vi "Select State(s)_err.vi"(0 "State(s) if True (\"\")":string, 5 "Select":errorcluster, 7 "State(s) if False (\"\")":string) -> (6 "States Out":string)   [LabVIEW 2013]
doc: "Passes State(s) based on a condition\n\nFor instructions on how to use the JKI State Machine, examples and video tutorials, visit:\nhttp://jkisoft.com/state-machine/"
panel:
  # "For instructions on how to use the JKI State Machine, examples and video tutorials, visit:\nhttp://jki.net/state-machine/\n\nJKI State Machine™\nhttp://jki.net/state-machine/\nCopyright (C) 2005-2024, JKI <info@jki.net>\nALL RIGHTS RESERVED"
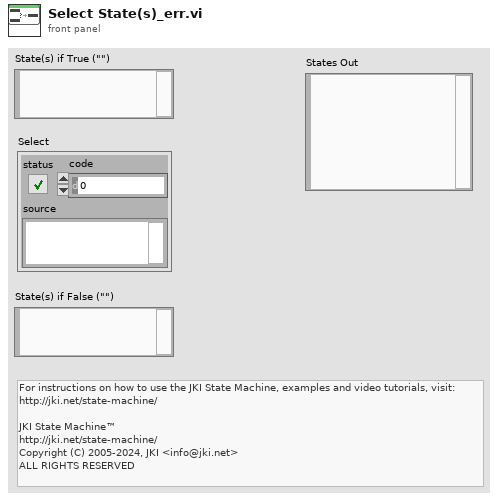
[diagram p1: front panel]
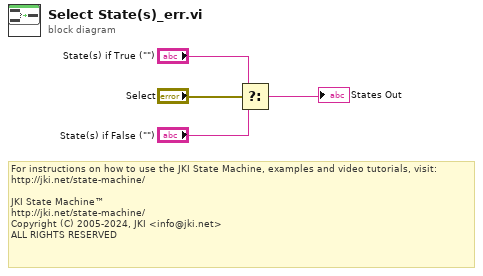
[diagram p0: block diagram]
diagram:
  # "For instructions on how to use the JKI State Machine, examples and video tutorials, visit:\nhttp://jki.net/state-machine/\n\nJKI State Machine™\nhttp://jki.net/state-machine/\nCopyright (C) 2005-2024, JKI <info@jki.net>\nALL RIGHTS RESERVED"
  n1 = Select(t="State(s) if True (\"\")", s="Select", f="State(s) if False (\"\")") -> (s? t:f=→"States Out":string)
